vi "HMF2500 Set Output State.vi"(8 "error in (no error)":errorcluster, 10 "Enabled (False)":bool, 11 "VISA in":refnum<visa-resource-name>) -> (0 "error out":errorcluster, 3 "VISA out":refnum<visa-resource-name>)   [LabVIEW 2020, in "AWG.lvlib"]
doc: "Set output state."
uses:
  AWG.lvlib
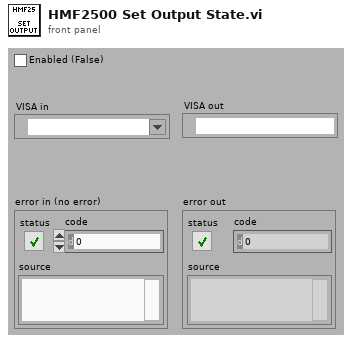
[diagram p1: front panel]
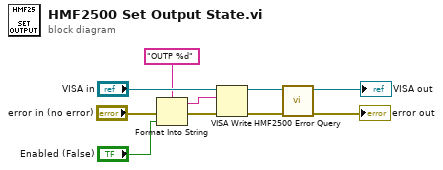
[diagram p0: block diagram]
diagram:
  n1 = Format Into String(format string="OUTP %d", error in="error in (no error)", "Enabled (False)") -> (resulting string=w8:string, error out=w9:errorcluster)  [unwired: 1 in]
  n2 = VISA Write(VISA resource name="VISA in", write buffer=w8, error in (no error)=w9) -> (VISA resource name out=w4:refnum<visa-resource-name>, error out=w5:errorcluster)  [unwired: 1 out]
  n3 = call "HMF2500 Error Query.vi"("error in (no error)"=w5, "VISA resource name"=w4) -> ("error out"=→"error out":errorcluster, "VISA resource name out"=→"VISA out":refnum<visa-resource-name>)  [unwired: 6 in, 2 out]
